vi "Update XNET Settings.vi"(10 "XNET Settings":T2, 11 "References":T1) -> ()   [LabVIEW 2015, in "J1939 editor node.lvclass"]
uses:
  J1939 editor node.lvclass
  module/configuration/XNET Settings.ctl
  <vilib>/NI/DCAF/Tag Editor Core/Table API/Table Manager/object ref.ctl
  <vilib>/NI/DCAF/Tag Editor Core/Configuration Editor/Classes/Engine Parent/Engine Parent Editor Node.lvclass
  <vilib>/NI/DCAF/Tag Editor Core/Configuration Editor/Classes/Module editor node/module editor node.lvclass
  module/configuration/J1939 configuration.lvclass
  module/configuration/J1939 configuration.lvclass/J1939 configuration.ctl
  module/configuration/Write XNET Settings.vi
  <vilib>/NI/Configuration Framework/serializable configuration/NISE_CEF_serializable configuration.lvclass
  <vilib>/NI/DCAF/Tag Editor Core/Table API/Table Manager/Table Manager.lvclass
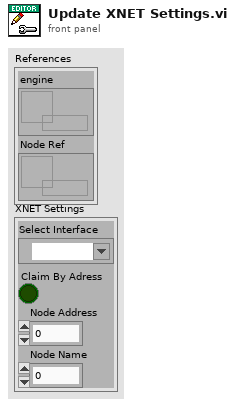
[diagram p1: front panel]
types:
  T1 = typedef "Table Manager.lvlib/Table Manager.lvclass/object ref.ctl" = cluster{"engine":refnum<data-value>, "Node Ref":refnum<data-value>}
  T2 = typedef "J1939 configuration.lvclass/XNET Settings.ctl" = cluster{"Select Interface":refnum<k21>, "Claim By Adress":bool, "Node Address":u8, "Node Name":u64}
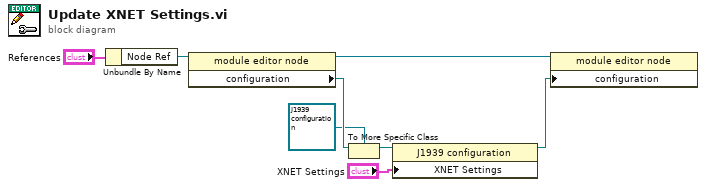
[diagram p0: block diagram]
diagram:
  n1 = Unbundle By Name("References") -> ("Node Ref"=w4:refnum<data-value>)
  n2 = property class="module editor node"(reference=w4) -> (reference out=w2:refnum<data-value>, "configuration"=w6:refnum<class "NISE_CEF_serializable configuration.lvclass">)  [unwired: 1 in, 1 out]
  n3 = To More Specific Class(target class=refnum<class "J1939 configuration.lvclass"> refnum ("J1939 configuration"), reference=w6) -> (specific class reference=w7:refnum<class "J1939 configuration.lvclass">)  [unwired: 1 in, 1 out]
  n4 = property class="J1939 configuration"(reference=w7, "XNET Settings"="XNET Settings") -> (reference out=w1:refnum<class "J1939 configuration.lvclass">)  [unwired: 1 in, 1 out]
  n5 = property class="module editor node"(reference=w2, "configuration"=w1) -> ()  [unwired: 1 in, 2 out]
